vi "Commit all build changes.vi"(8 "error in":errorcluster, 11 "msg":string="Automatically generated commit") -> (0 "error out":errorcluster, 3 "appended array":string[](array[string]))   [LabVIEW 2021]
uses:
  <vilib>/Hampel Software Engineering/Git API/Git API/GIT-api.lvclass/GIT-api.ctl
  <vilib>/Hampel Software Engineering/Git API/Git API/Accessors/GIT-Set Working Dir.vi
  <vilib>/Hampel Software Engineering/Git API/Git API/GIT-api.lvclass
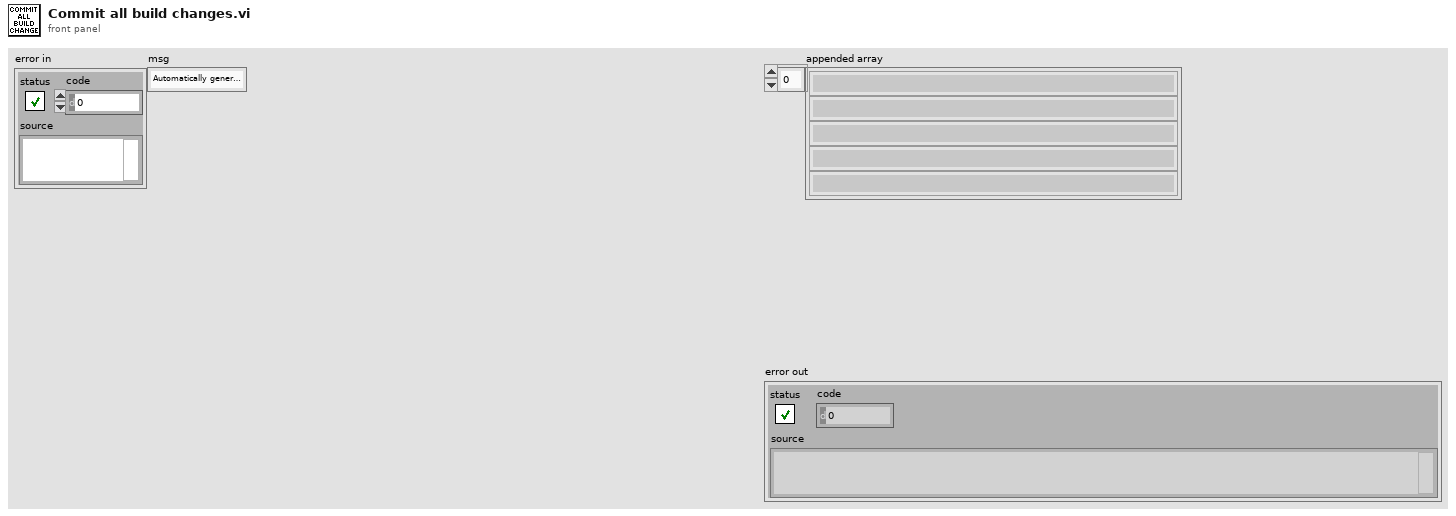
[diagram p1: front panel]
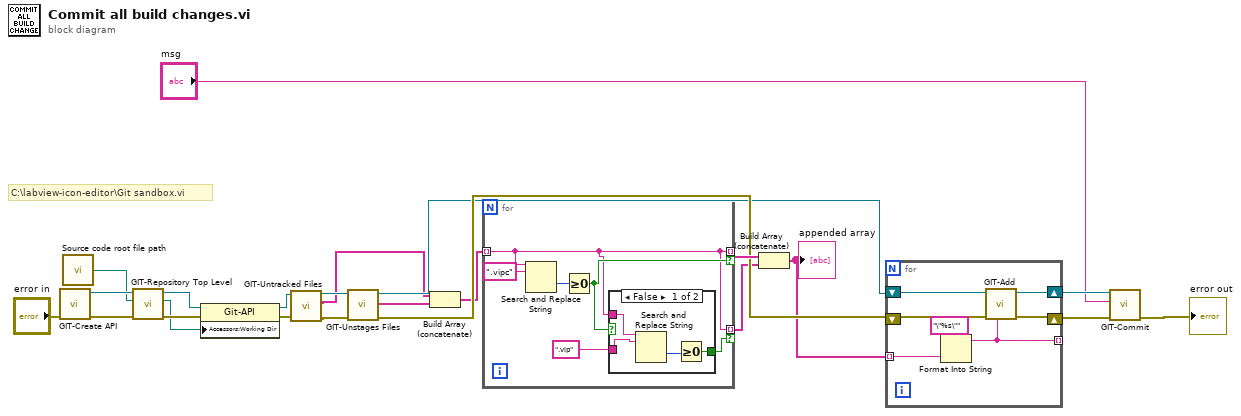
[diagram p0: block diagram]
diagram:
  # "C:\\labview-icon-editor\\Git sandbox.vi"
  n1 = call <vilib>:"GIT-Create API.vi"("error in"="error in") -> ("error out"=w20:errorcluster, "git-api out"=w22:refnum<class "GIT-api.lvclass">)  [unwired: 9 in]
  n2 = call "Source code root file path.vi"() -> ("Source code root path"=w19:path)  [unwired: 1 in]
  n3 = call <vilib>:"GIT-Repository Top Level.vi"("error in"=w20, "Current Path"=w19, "git-api in"=w22) -> ("error out"=w21:errorcluster, "Repo Top Level Path"=w18:path, "git-api out"=w23:refnum<class "GIT-api.lvclass">)  [unwired: 6 in]
  n4 = property class="Git-API"(reference=w23, error in=w21, "Accessors:Working Dir"=w18) -> (reference out=w14:refnum<class "GIT-api.lvclass">, error out=w15:errorcluster)
  n5 = call <vilib>:"GIT-Untracked Files.vi"("error in"=w15, "Git-API in"=w14) -> ("error out"=w13:errorcluster, "Untracked Files"=w6:string[], "Git-API out"=w12:refnum<class "GIT-api.lvclass">)  [unwired: 7 in]
  n6 = call <vilib>:"GIT-Unstages Files.vi"("error in"=w13, "Git-API in"=w12) -> ("error out"=w11:errorcluster, "Unstaged Files"=w7:string[], "Git-API out"=w10:refnum<class "GIT-api.lvclass">)  [unwired: 7 in]
  n7 = Build Array (concatenate)(w6, w7) -> (w5:string[])
  n8 = for {
    tunnel: w5 -> [w25] mode=indexing
    tunnel: [w25] -> w17 mode=indexing if=w27
    tunnel: [w25] -> w8 mode=indexing if=w24
    n9 = Search and Replace String(input string=w25, search string=".vipc") -> (offset past replacement=w28:i32)  [unwired: 6 in, 3 out]
    n10 = Greater Or Equal To 0?(x=w28) -> (x >= 0?=w27:bool)
    n11 = case shown="False" w27 {
      tunnel: w25 -> [w33 _]
      tunnel: ".vip" ("search string") -> [w32 _]
      tunnel: [w30 _] -> w24
      frame False {
        n12 = Search and Replace String(input string=w33, search string=w32) -> (offset past replacement=w31:i32)  [unwired: 6 in, 3 out]
        n13 = Greater Or Equal To 0?(x=w31) -> (x >= 0?=w30:bool)
      }
      frame True {
      }
    }
  }
  n14 = Build Array (concatenate)(w17, w8) -> (w9:string[])
  "appended array" <- w9
  n15 = for {
    tunnel: w9 -> [w36] mode=indexing
    shift-right: [w38] -> w4
    shift-left: w10 -> [w39]
    shift-right: [w37] -> w3
    shift-left: w11 -> [w40]
    tunnel: [w34] -> _ mode=indexing
    n16 = Format Into String(format string="\"%s\"", w36) -> (resulting string=w34:string)  [unwired: 2 in, 1 out]
    n17 = call <vilib>:"GIT-Add.vi"("param"=w34, "error in"=w40, "git-api in"=w39) -> ("error out"=w37:errorcluster, "git-api out"=w38:refnum<class "GIT-api.lvclass">)  [unwired: 6 in, 1 out]
  }
  n18 = call <vilib>:"GIT-Commit.vi"("error in"=w3, "msg"="msg", "Git-API in"=w4) -> ("error out"=→"error out":errorcluster)  [unwired: 7 in, 1 out]
